vi "HelloWorldInCv.vi"   [LabVIEW 2018]
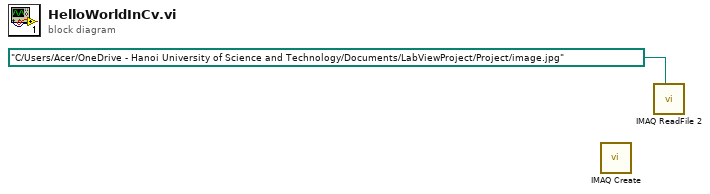
[diagram p0: block diagram]
diagram:
  n1 = call "IMAQ Create"() -> ()  [unwired: 5 in, 2 out]
  n2 = call "IMAQ ReadFile 2"("File Path"=path "C:/Users/Acer/OneDrive - Hanoi University of Science and Technology/Documents/LabViewProject/Project/image.jpg") -> ()  [unwired: 6 in, 5 out]
